vi "GetTypes.vi"(0 "vi reference":refnum<vi>, 1 "controls or indicators":cluster{"Name":string, "Variant Data":variant}[](array[cluster])) -> (7 "types":T1(array[cluster]))   [LabVIEW 2019]
uses:
  <vilib>/Utility/VariantDataType/VariantType.lvlib
panel:
  # "Get All Types"
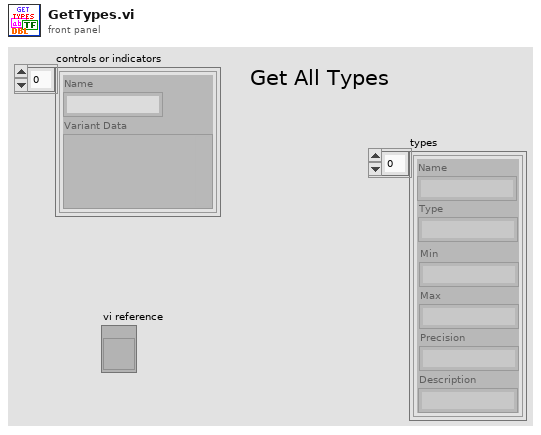
[diagram p1: front panel]
types:
  T1 = cluster{"Name":string, "Type":string, "Min":string, "Max":string, "Precision":string, "Description":string}[]
  T2 = cluster{"Name":string, "Type":string, "Min":string, "Max":string, "Precision":string, "Description":string}
  T3 = typedef "VariantType.lvlib/Type.ctl" = enum8{"Invalid Type", "Void", "I8", "I16", "I32", "I64", "U8", "U16", "U32", "U64", "Single Float", "Double Float", "Extended Float", "Single Complex", "Double Complex", "Extended Complex", "Enum U8", "Enum U16", "Enum U32", "Enum U64", "Single Float With Unit", "Double Float With Unit", "Extended Float With Unit", "Single Complex with Unit", "Double Complex with Unit", "Extended Complex with Unit", "Boolean", "String", "Path", "Picture", "Tag", "Array", "Cluster", "Variant", "LV Variant", "Waveform", "Timestamp", "Digital Waveform", "Digital Data", "ExpressData", "Refnum", "External Data", "VI", "Poly VI", "LabVIEW Class Instance", "Fixed Point"}
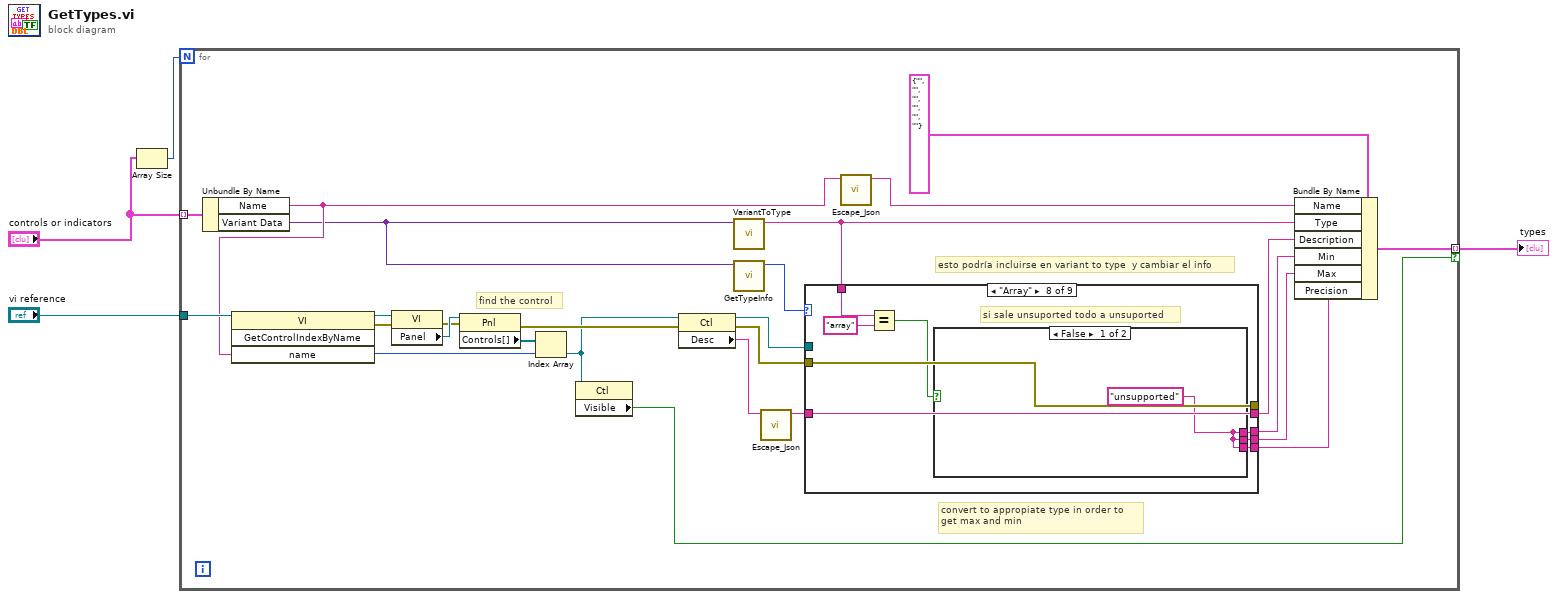
[diagram p0: block diagram]
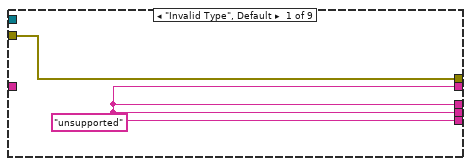
[diagram p2: hidden frame]
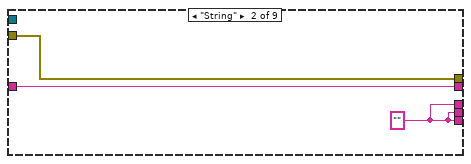
[diagram p3: hidden frame]
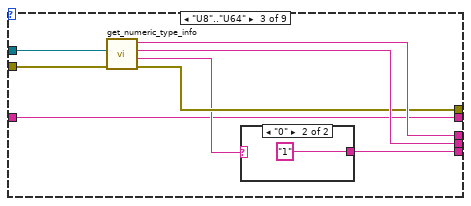
[diagram p4: hidden frame]
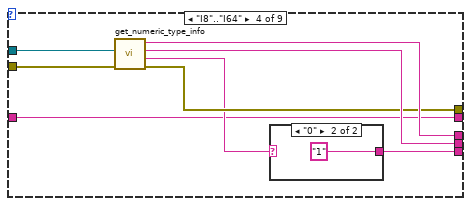
[diagram p6: hidden frame]
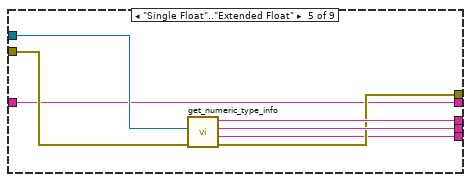
[diagram p8: hidden frame]
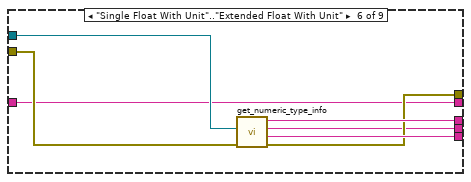
[diagram p9: hidden frame]
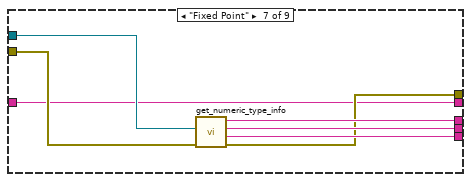
[diagram p10: hidden frame]
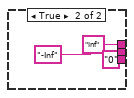
[diagram p11: hidden frame]
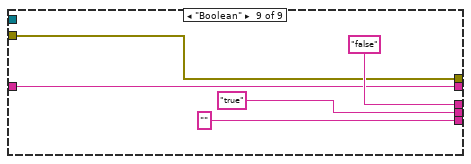
[diagram p12: hidden frame]
diagram:
  n1 = Array Size(array="controls or indicators") -> (size(s)=w4:i32)
  n2 = for {
    N: w4 -> [_]
    tunnel: "controls or indicators" -> [w30] mode=indexing
    tunnel: "vi reference" -> [w29]
    tunnel: [w19] -> w3 mode=indexing if=w8
    # "esto podría incluirse en variant to type  y cambiar el info"
    # "convert to appropiate type in order to \nget max and min"
    # "find the control"
    n3 = Unbundle By Name(w30) -> ("Name"=w21:string, "Variant Data"=w6:variant)
    n4 = invoke class="VI" method="GetControlIndexByName"(reference=w29, "name"=w21) -> (reference out=w28:refnum<vi>, error out=w24:errorcluster, "GetControlIndexByName"=w26:i32)  [unwired: 2 in, 1 out]
    n5 = property class="VI"(reference=w28, error in=w24) -> (error out=w23:errorcluster, "Panel"=w27:refnum<vi>)  [unwired: 1 out]
    n6 = property class="Pnl"(reference=w27, error in=w23) -> (error out=w22:errorcluster, "Controls[]"=w25:refnum<vi>[])  [unwired: 1 out]
    n7 = Index Array(array=w25, index=w26) -> (element=w20:refnum<vi>)
    n8 = property class="Ctl"(reference=w20) -> ("Visible"=w8:bool)  [unwired: 1 in, 2 out]
    n9 = property class="Ctl"(reference=w20, error in=w22) -> (reference out=w16:refnum<vi>, error out=w17:errorcluster, "Desc"=w12:string)
    n10 = call "VariantToType.vi"("Variant"=w6) -> ("type Name"=w5:string)  [unwired: 10 in]
    n11 = call <vilib>:"GetTypeInfo.vi"("Variant"=w6) -> ("Type Enum"=w7:T3)  [unwired: 6 in, 4 out]
    n12 = call "Escape_Json.vi"("String"=w12) -> ("Json_string"=w11:string)  [unwired: 9 in]
    n13 = case shown="\"Array\"" w7 {
      tunnel: [w31 w35 w37 w47 w57 w68 w74 w84 ""] -> w9
      tunnel: [w31 w35 w42 w52 w61 w63 w75 w83 "true"] -> w14
      tunnel: [w31 w35 w43 w53 w62 w69 w76 w82 "false"] -> w15
      tunnel: [w32 w34 w41 w51 w60 w67 w73 w80 w90] -> _
      tunnel: w17 -> [w32 w34 w40 w49 w59 w65 w72 w80 w90]
      tunnel: w16 -> [_ _ w39 w50 w58 w66 w71 _ _]
      tunnel: w11 -> [_ w33 w36 w46 w56 w64 w70 w81 w89]
      tunnel: [w31 w33 w36 w46 w56 w64 w70 w81 w89] -> w13
      tunnel: w5 -> [_ _ _ _ _ _ _ w79 _]
      frame "Invalid Type", Default {
        w31 = "unsupported"
      }
      frame "String" {
        w35 = "" ("Min")
      }
      frame "U8".."U64" {
        n14 = call "get_numeric_type_info.vi"("error in (no error)"=w40, "Refnum"=w39) -> ("error out"=w41:errorcluster, "Precision"=w38:string, "max"=w42:string, "Min"=w43:string)  [unwired: 6 in]
        n15 = case shown="\"0\"" w38 {
          selector: w38 -> [w44 _]
          tunnel: [w44 "1" ("Precision")] -> w37
          frame "False", Default {
          }
          frame "0" {
          }
        }
      }
      frame "I8".."I64" {
        n16 = call "get_numeric_type_info.vi"("error in (no error)"=w49, "Refnum"=w50) -> ("error out"=w51:errorcluster, "Precision"=w48:string, "max"=w52:string, "Min"=w53:string)  [unwired: 6 in]
        n17 = case shown="\"0\"" w48 {
          selector: w48 -> [w54 _]
          tunnel: [w54 "1" ("Precision")] -> w47
          frame "False", Default {
          }
          frame "0" {
          }
        }
      }
      frame "Single Float".."Extended Float" {
        n18 = call "get_numeric_type_info.vi"("error in (no error)"=w59, "Refnum"=w58) -> ("error out"=w60:errorcluster, "Precision"=w57:string, "max"=w61:string, "Min"=w62:string)  [unwired: 6 in]
      }
      frame "Single Float With Unit".."Extended Float With Unit" {
        n19 = call "get_numeric_type_info.vi"("error in (no error)"=w65, "Refnum"=w66) -> ("error out"=w67:errorcluster, "Precision"=w68:string, "max"=w63:string, "Min"=w69:string)  [unwired: 6 in]
      }
      frame "Fixed Point" {
        n20 = call "get_numeric_type_info.vi"("error in (no error)"=w72, "Refnum"=w71) -> ("error out"=w73:errorcluster, "Precision"=w74:string, "max"=w75:string, "Min"=w76:string)  [unwired: 6 in]
      }
      frame "Array" {
        # "si sale unsuported todo a unsuported"
        n21 = Equal?(x=w79, y="array") -> (x = y?=w77:bool)
        n22 = case shown="False" w77 {
          tunnel: [w85 "0" ("Precision")] -> w84
          tunnel: [w85 "-Inf" ("max")] -> w83
          tunnel: [w85 "Inf" ("Min")] -> w82
          frame False {
            w85 = "unsupported" ("Min")
          }
          frame True {
          }
        }
      }
      frame "Boolean" {
      }
    }
    n23 = call "Escape_Json.vi"("String"=w21) -> ("Json_string"=w10:string)  [unwired: 9 in]
    n24 = Bundle By Name(cluster=T2 {"Name"="", "Type"="", "Min"="", "Max"="", "Precision"="", "Description"=""} ("element"), "Name"=w10, "Type"=w5, "Description"=w13, "Min"=w15, "Max"=w14, "Precision"=w9) -> (w19:T2)
  }
  "types" <- w3
